vi "oldBallToOOBall.vi"(8 "error in (no error)":errorcluster, 10 "balls":T1[](array[typedef]), 11 "Ball in":refnum<class "Ball.lvclass">) -> (0 "error out":errorcluster, 3 "Ball out":refnum<class "Ball.lvclass">)   [LabVIEW 2023, in "Ball.lvclass"]
uses:
  Ball.lvclass
  Vision_class/Old vision/SSL Detection Frame Simple Estimator Cameras VelCmd Folder/Core/AI Ball.ctl
  Object_class/Object.lvclass/Object.ctl
  Ball.lvclass/Ball.ctl
  Object_class/Write x.vi
  Object_class/Write y.vi
  Write v_x.vi
  Write v_y.vi
  Object_class/Write pos_est_x.vi
  Object_class/Write pos_est_y.vi
  Write Valid.vi
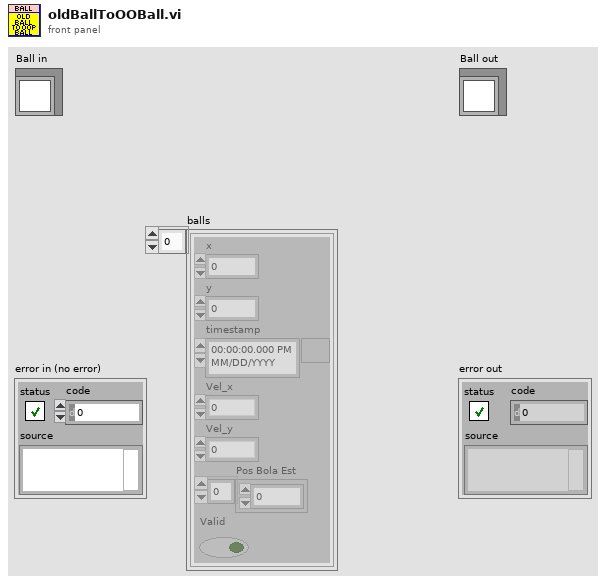
[diagram p1: front panel]
types:
  T1 = typedef "AI Ball.ctl" = cluster{"x":dbl, "y":dbl, "timestamp":timestamp, "Vel_x":dbl, "Vel_y":dbl, "Pos Bola Est":dbl[], "Valid":bool}
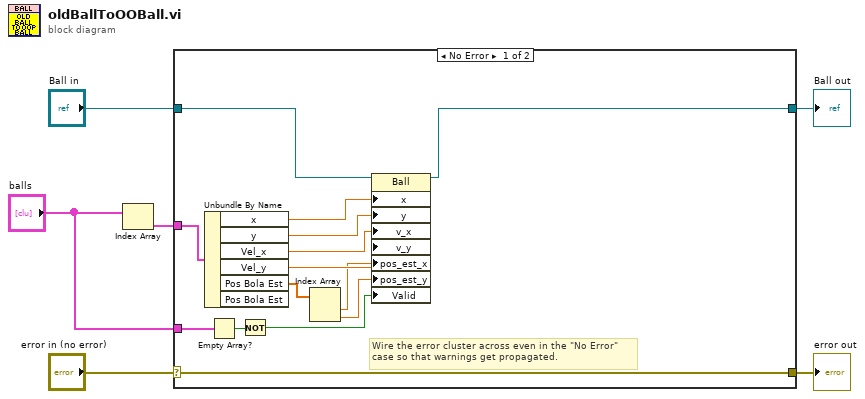
[diagram p0: block diagram]
diagram:
  n1 = Index Array(array="balls") -> (element=w2:T1)  [unwired: 1 in]
  n2 = case shown="No Error" "error in (no error)" {
    selector: "error in (no error)" -> [w20 w22]
    tunnel: [w20 w22] -> w5
    tunnel: [w15 w21] -> w3
    tunnel: "Ball in" -> [w19 w21]
    tunnel: w2 -> [w18 _]
    tunnel: "balls" -> [w9 _]
    frame No Error {
      # "Wire the error cluster across even in the \"No Error\"\ncase so that warnings get propagated."
      n3 = Unbundle By Name(w18) -> ("x"=w17:dbl, "y"=w16:dbl, "Vel_x"=w14:dbl, "Vel_y"=w13:dbl, "Pos Bola Est"=w12:dbl[])  [unwired: 1 out]
      n4 = Empty Array?(array=w9) -> (empty?=w8:bool)
      n5 = Not(x=w8) -> (.not. x?=w7:bool)
      n6 = Index Array(array=w12) -> (element #1=w11:dbl, element #2=w10:dbl)  [unwired: 2 in]
      n7 = property class="Ball"(reference=w19, "x"=w17, "y"=w16, "v_x"=w14, "v_y"=w13, "pos_est_x"=w11, "pos_est_y"=w10, "Valid"=w7) -> (reference out=w15:refnum<class "Ball.lvclass">)  [unwired: 1 in, 1 out]
    }
    frame Error {
    }
  }
  "error out" <- w5
  "Ball out" <- w3
